vi "Sensors.vi"(0 "AIDeviceRef":T4, 1 "GyroDevRef":T7, 2 "Aquisition Sensor":T1, 3 "BottomAquistion 2":T1, 5 "BottomAquistion":T1) -> ()   [LabVIEW 2014]
uses:
  <vilib>/Rock Robotics/WPI/Gyro/WPI_GyroDevRef.ctl
  <vilib>/Rock Robotics/SystemInterfaces/Typedef/FPGA_TypedefAnalogModule.ctl
  <vilib>/Rock Robotics/SystemInterfaces/AI/FPGA_AIChannel.ctl
  <vilib>/Rock Robotics/WPI/DigitalInput/WPI_DigitalInputDevRef.ctl
  <vilib>/Rock Robotics/SystemInterfaces/DIO/FPGA_DIOChannel.ctl
  <vilib>/Rock Robotics/SystemInterfaces/Typedef/FPGA_TypedefDigitalModule.ctl
  <vilib>/Rock Robotics/WPI/AnalogChannel/WPI_AnalogChannelDevRef.ctl
  Events.vi
panel:
  in  "test":bool
  out "Angular Rate":dbl
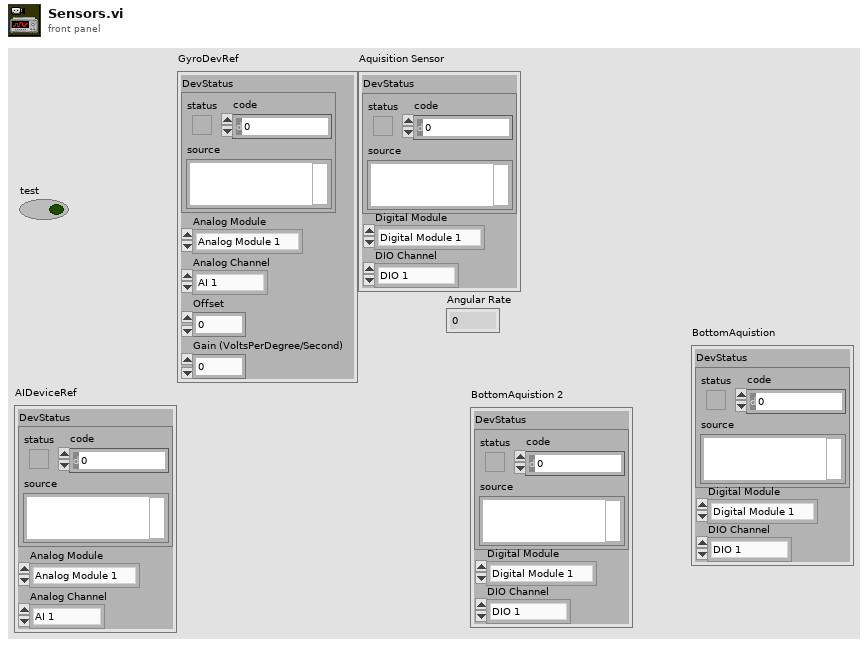
[diagram p1: front panel]
types:
  T1 = typedef "WPI_DigitalInputDevRef.ctl" = cluster{"DevStatus":errorcluster, "DIO Channel":T2, "Digital Module":T3}
  T2 = typedef "FPGA_DIOChannel.ctl" = enum8{"DIO 1", "DIO 2", "DIO 3", "DIO 4", "DIO 5", "DIO 6", "DIO 7", "DIO 8", "DIO 9", "DIO 10", "DIO 11", "DIO 12", "DIO 13", "DIO 14", "Invalid"}
  T3 = typedef "FPGA_TypedefDigitalModule.ctl" = enum16{"Digital Module 1", "Digital Module 2"}
  T4 = typedef "WPI_AnalogChannelDevRef.ctl" = cluster{"DevStatus":errorcluster, "Analog Module":T5, "Analog Channel":T6}
  T5 = typedef "FPGA_TypedefAnalogModule.ctl" = enum16{"Analog Module 1", "Analog Module 2"}
  T6 = typedef "FPGA_AIChannel.ctl" = enum8{"AI 1", "AI 2", "AI 3", "AI 4", "AI 5", "AI 6", "AI 7", "AI 8", "Invalid"}
  T7 = typedef "WPI_GyroDevRef.ctl" = cluster{"DevStatus":errorcluster, "Analog Module":T5, "Analog Channel":T6, "Offset":dbl, "Gain (VoltsPerDegree/Second)":dbl}
  T8 = typedef "WPI_SolenoidValue.ctl" = enum16{"Off", "On", "Forward", "Reverse"}
  T9 = cluster{"Ultrasonic Distance (In)":dbl, "Gyro":dbl, "TopAquisition sensor":bool, "Encoder distance":dbl, "Encoder rate":dbl, "Encoder direction":bool, "winch engaged?":T8, "Motor Values":dbl[], "Latch encoder":u32, "BottomAquistion":bool, "BottomAquistion 2":bool, "Gyro Rate":dbl}
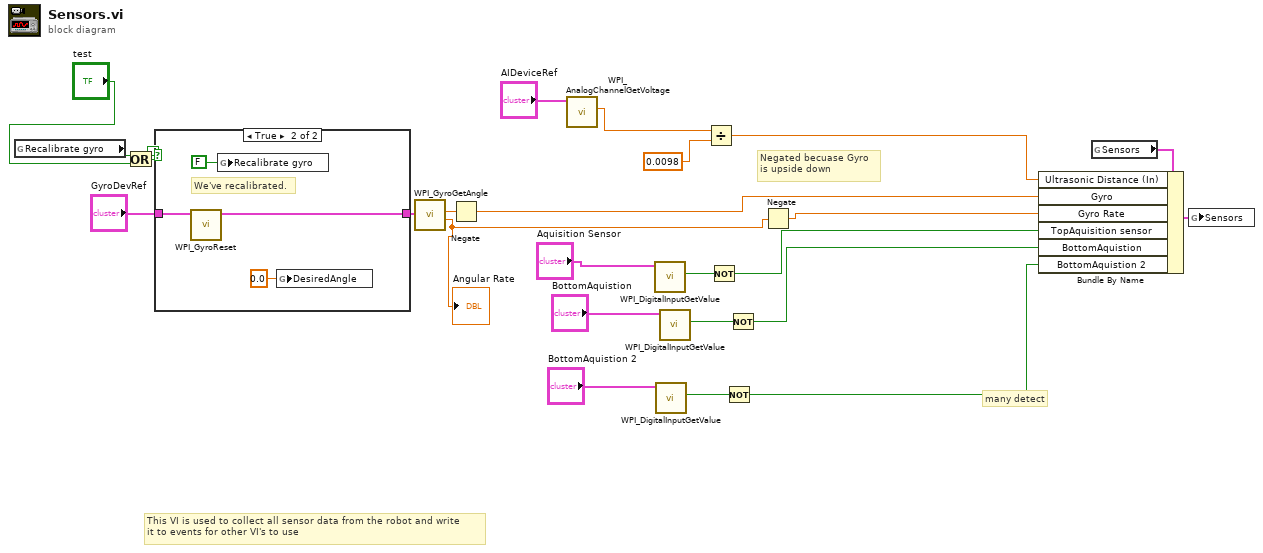
[diagram p0: block diagram]
diagram:
  # "Negated becuase Gyro\nis upside down"
  # "This VI is used to collect all sensor data from the robot and write\nit to events for other VI's to use"
  # "many detect"
  n1 = global read "Events.vi" "Recalibrate gyro"() -> (w18:bool)
  n2 = Or(x=w18, y="test") -> (x .or. y?=w9:bool)
  n3 = case shown="True" w9 {
    tunnel: [w25 w28] -> w22
    tunnel: "GyroDevRef" -> [w25 w29]
    frame False {
    }
    frame True {
      # "We've recalibrated."
      n4 = call <vilib>:"WPI_GyroReset.vi"("GyroDevRef"=w29) -> ("GyroDevRef"=w28:T7)  [unwired: 9 in, 1 out]
      n5 = global write "Events.vi" "Recalibrate gyro"(FALSE) -> ()
      n6 = global write "Events.vi" "DesiredAngle"(0.0 ("DesiredAngle")) -> ()
    }
  }
  n7 = call <vilib>:"WPI_GyroGetAngle.vi"("GyroDevRef"=w22) -> ("Angular Rate"=w3:dbl, "Angle"=w4:dbl)  [unwired: 7 in, 2 out]
  "Angular Rate" <- w3
  n8 = Negate(x=w4) -> (-x=w2:dbl)
  n9 = call <vilib>:"WPI_AnalogChannelGetVoltage.vi"("AIDeviceRef"="AIDeviceRef") -> ("Voltage"=w11:dbl)  [unwired: 8 in, 2 out]
  n10 = call <vilib>:"WPI_DigitalInputGetValue.vi"("DigitalInputDevRef"="Aquisition Sensor") -> ("Value"=w19:bool)  [unwired: 8 in, 2 out]
  n11 = call <vilib>:"WPI_DigitalInputGetValue.vi"("DigitalInputDevRef"="BottomAquistion 2") -> ("Value"=w7:bool)  [unwired: 8 in, 2 out]
  n12 = call <vilib>:"WPI_DigitalInputGetValue.vi"("DigitalInputDevRef"="BottomAquistion") -> ("Value"=w17:bool)  [unwired: 8 in, 2 out]
  n13 = Divide(x=w11, y=0.0098) -> (x/y=w12:dbl)
  n14 = Not(x=w19) -> (.not. x?=w14:bool)
  n15 = Not(x=w7) -> (.not. x?=w5:bool)
  n16 = Not(x=w17) -> (.not. x?=w15:bool)
  n17 = Negate(x=w3) -> (-x=w1:dbl)
  n18 = global read "Events.vi" "Sensors"() -> (w23:T9)
  n19 = Bundle By Name(cluster=w23, "Ultrasonic Distance (In)"=w12, "Gyro"=w2, "Gyro Rate"=w1, "TopAquisition sensor"=w14, "BottomAquistion"=w15, "BottomAquistion 2"=w5) -> (w24:T9)
  n20 = global write "Events.vi" "Sensors"(w24) -> ()
